vi "SetCol.vi"(4 "ModeCol Index":i32=2, 5 "Col Array Ref in":refnum<vi>, 6 "Cell Position":T1, 7 "Table History ref":refnum<vi>, 8 "error in (no error)":errorcluster, 9 "Table CtlRef In":refnum<vi>, 10 "SetTo":string, 11 "MenuCol in":refnum<class "MenuCol.lvclass">) -> (0 "error out":errorcluster, 1 "Table CtlRef Out":refnum<vi>, 2 "Num Rows":i32, 3 "MenuCol out":refnum<class "MenuCol.lvclass">)   [LabVIEW 2013, in "MenuCol.lvclass"]
uses:
  MenuCol.lvclass
  <vilib>/Utility/miscctls.llb/LVRowAndColumnTypeDef.ctl
  TypeDefs/TableHistory.ctl
  TypeDefs/TableArray.ctl
  Column/Column.lvclass/Column.ctl
  Column/Column.lvclass
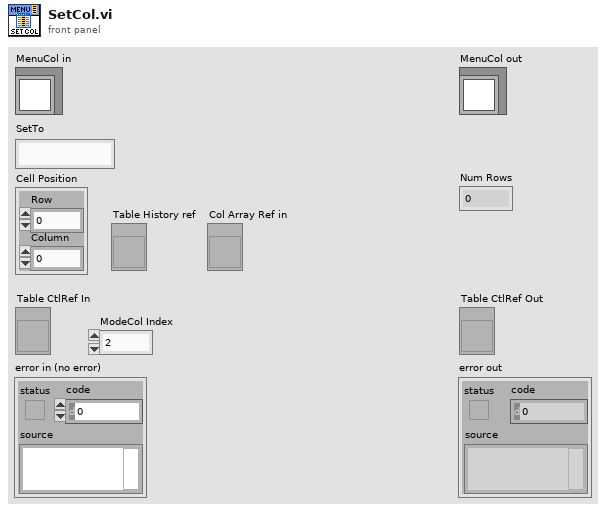
[diagram p1: front panel]
types:
  T1 = typedef "LVRowAndColumnTypeDef.ctl" = cluster{"Row":i32, "Column":i32}
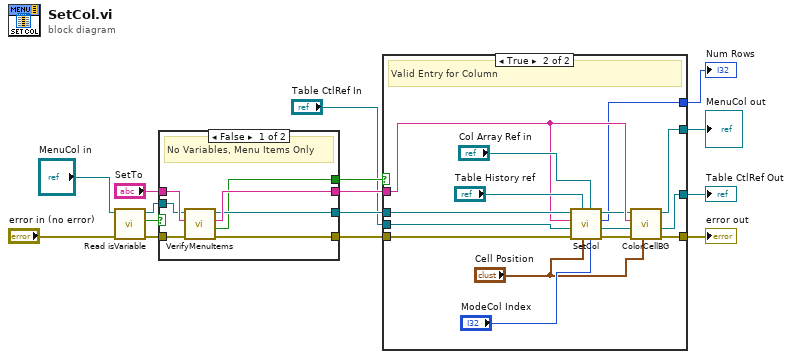
[diagram p0: block diagram]
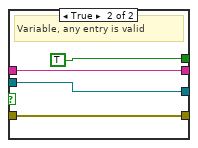
[diagram p2: hidden frame]
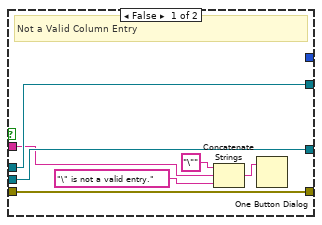
[diagram p3: hidden frame]
diagram:
  n1 = call "Read isVariable.vi"("error in (no error)"="error in (no error)", "Column in"="MenuCol in") -> ("error out"=w3:errorcluster, "isVariable?"=w2:bool, "Column out"=w5:refnum<class "MenuCol.lvclass">)  [unwired: 7 in]
  n2 = case shown="False" w2 {
    tunnel: "SetTo" -> [w22 w23]
    tunnel: [w21 w23] -> w14
    tunnel: [w20 w25] -> w13
    tunnel: [w19 w24] -> w12
    tunnel: [w18 TRUE ("Unknown Menu Item")] -> w11
    tunnel: w5 -> [w17 w25]
    tunnel: w3 -> [w16 w24]
    frame False {
      # "No Variables, Menu Items Only"
      n3 = call-dynamic "VerifyMenuItems.vi"("error in (no error)"=w16, "Menu Item In"=w22, "MenuCol in"=w17) -> ("error out"=w19:errorcluster, "Valid Menu Item"=w18:bool, "Menu Item Out"=w21:string, "MenuCol out"=w20:refnum<class "MenuCol.lvclass">)  [unwired: 5 in]
    }
    frame True {
      # "Variable, any entry is valid"
    }
  }
  n4 = case shown="True" w11 {
    tunnel: w14 -> [w27 w39]
    tunnel: w13 -> [w33 w45]
    tunnel: w12 -> [w31 w44]
    tunnel: [w31 w42] -> w10
    tunnel: [w32 w35] -> w9
    tunnel: [_ w34] -> w8
    tunnel: [w33 w36] -> w7
    tunnel: "Table CtlRef In" -> [w32 w43]
    frame False {
      # "Not a Valid Column Entry"
      n5 = Concatenate Strings("\"" ("string"), w27, "\" is not a valid entry." ("string")) -> (w30:string)
      n6 = One Button Dialog(message=w30) -> ()  [unwired: 1 in, 1 out]
    }
    frame True {
      # "Valid Entry for Column"
      n7 = call-parent "SetCol.vi"("ModeCol Index"="ModeCol Index", "Col Array Ref in"="Col Array Ref in", "Cell Position"="Cell Position", "Table History ref"="Table History ref", "error in (no error)"=w44, "Table CtlRef In"=w43, "SetTo"=w39, "Column in"=w45) -> ("error out"=w41:errorcluster, "Table CtlRef Out"=w38:refnum<vi>, "Num Rows"=w34:i32, "Column out"=w37:refnum<class "MenuCol.lvclass">)
      n8 = call-dynamic "ColorCellBG.vi"("Cell Position"="Cell Position", "error in (no error)"=w41, "Table CtlRef In"=w38, "Value"=w39, "MenuCol in"=w37) -> ("error out"=w42:errorcluster, "Table CtlRef Out"=w35:refnum<vi>, "MenuCol out"=w36:refnum<class "MenuCol.lvclass">)  [unwired: 4 in]
    }
  }
  "MenuCol out" <- w7
  "Num Rows" <- w8
  "Table CtlRef Out" <- w9
  "error out" <- w10
